vi "MTM2_monitorCommand_applyForce.vi"(8 "error in (no error)":errorcluster, 11 "command_applyForce_Ctl":T1={"forceSetPoint[72]"=[0.0, 0.0, 0.0, 0.0, 0.0, 0.0, 0.0, 0.0, 0.0, 0.0, 0.0, 0.0, 0.0, 0.0, 0.0, 0.0, 0.0, 0.0, 0.0, 0.0, 0.0, 0.0, 0.0, 0.0, 0.0, 0.0, 0.0, 0.0, 0.0, 0.0, 0.0, 0.0, 0.0, 0.0, 0.0, 0.0, 0.0, 0.0, 0.0, 0.0, 0.0, 0.0, 0.0, 0.0, 0.0, 0.0, 0.0, 0.0, 0.0, 0.0, 0.0, 0.0, 0.0, 0.0, 0.0, 0.0, 0.0, 0.0, 0.0, 0.0, 0.0, 0.0, 0.0, 0.0, 0.0, 0.0, 0.0, 0.0, 0.0, 0.0, 0.0, 0.0]}) -> (0 "error out":errorcluster, 2 "function return":i32, 3 "command_applyForce_Ctl out":T1)   [LabVIEW 2018, in "SALLV_MTM2.lvlib"]
doc: "int MTM2_shm_monitorCommand_applyForceLV(MTM2_command_applyForceLV *command_applyForce_Ctl );"
uses:
  SALLV_MTM2.lvlib
  DataTypes/command_applyForce.ctl
  SALLV_MTM2.so
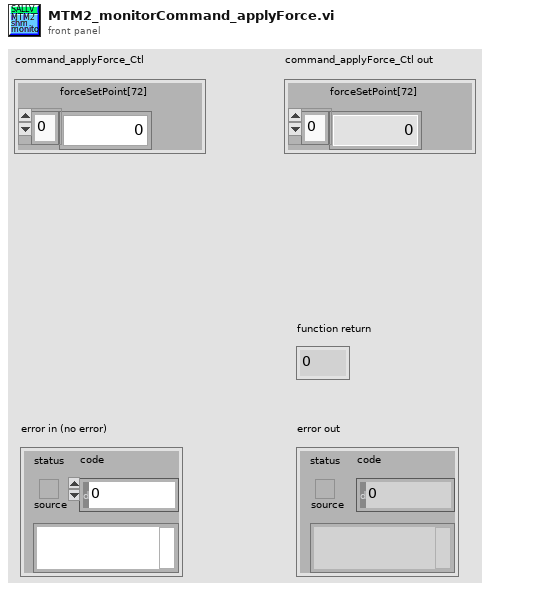
[diagram p1: front panel]
types:
  T1 = typedef "SALLV_MTM2.lvlib/command_applyForce.ctl" = cluster{"forceSetPoint[72]":dbl[]}
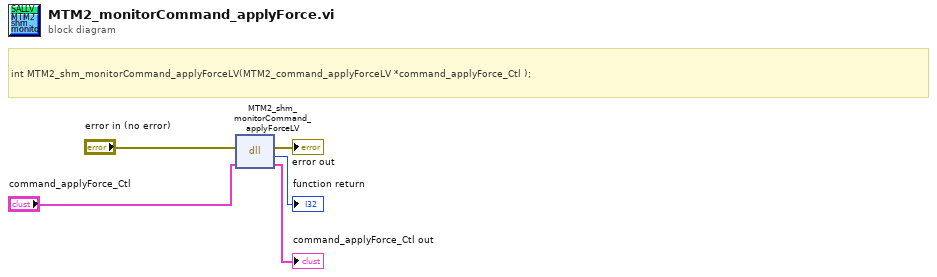
[diagram p0: block diagram]
diagram:
  # "int MTM2_shm_monitorCommand_applyForceLV(MTM2_command_applyForceLV *command_applyForce_Ctl );"
  n1 = dll-call lib="home/ttsai/Document/salApiMTM2/SALLV_MTM2/SALLV_MTM2.*" fn="MTM2_shm_monitorCommand_applyForceLV"(error in="error in (no error)", "command_applyForce_Ctl"="command_applyForce_Ctl") -> (error out=→"error out":errorcluster, →"function return":i32, "command_applyForce_Ctl"=→"command_applyForce_Ctl out":T1)  [unwired: 2 in, 1 out]
